vi "Waveform simulator.vi"(1 "Waveform Parameters":T1) -> ()   [LabVIEW 2015]
uses:
  <vilib>/imath/engines/lvmath2/RunTimeEngine/Managers/WorkSpace/UID Generator.vi
  <vilib>/imath/engines/lvmath2/RunTimeEngine/LocalVariableDefStatement/MC_LocalVariableDefStatement_Display.vi
  <vilib>/imath/engines/lvmath2/RunTimeEngine/RunTimeType/NIMS_RunTimeType_From StrictType (excl LVString).vi
  <vilib>/imath/engines/lvmath2/RunTimeEngine/RangeToken/NIMS_Range.vi
  <vilib>/imathl/engines/lvmath/Functions/Error Handling/Create Error.vi
  <vilib>/imath/engines/lvmath2/RunTimeEngine/BuiltInFunctions/linramp/NIMS_linramp.vi
  <vilib>/imath/engines/lvmath2/RunTimeEngine/BuiltInFunctions/gensignal/NIMS_gensignal(str,RS,RS,RS).vi
  <vilib>/imath/engines/lvmath2/RunTimeEngine/BuiltInFunctions/transpose/NIMS_transpose(GV).vi
  <vilib>/imath/engines/lvmath2/RunTimeEngine/ArithmeticOperatorToken/NIMS_ArithmeticOperator_plus.vi
  <vilib>/imath/engines/lvmath2/RunTimeEngine/VariableToken/NIMS_VariableToken_CondDefined.vi
  <vilib>/imath/engines/lvmath2/RunTimeEngine/Managers/SymbolTable/Clear UID.vi
  <vilib>/imath/engines/lvmath2/RunTimeEngine/Managers/SymbolTable/NIMS_WorkSpace.lvlib
  <vilib>/imath/engines/lvmath/Functions/Error Handling/MergeErrorsWrapper.vi
  <vilib>/imath/engines/lvmath2/RunTimeEngine/NodeEndStatement/NIMS_NodeEndStatement_Output.vi
  <vilib>/imath/engines/lvmath2/RunTimeEngine/ErrorHandling/NIMS_Finalize Error.vi
panel:
  in  "Digitizing Parameters":T2
  out "XY Graph":cluster{"t":dbl[], "x":dbl[]}(graph)
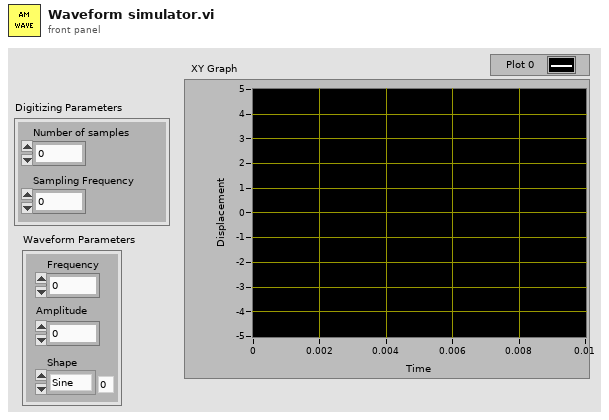
[diagram p1: front panel]
types:
  T1 = cluster{"Frequency":dbl, "Amplitude":dbl, "Shape":enum16{"Sine", "Cosine", "DC Level", "Square", "User Defined"}}
  T2 = cluster{"Number of samples":dbl, "Sampling Frequency":dbl}
  T3 = enum16{"Sine", "Cosine", "DC Level", "Square", "User Defined"}
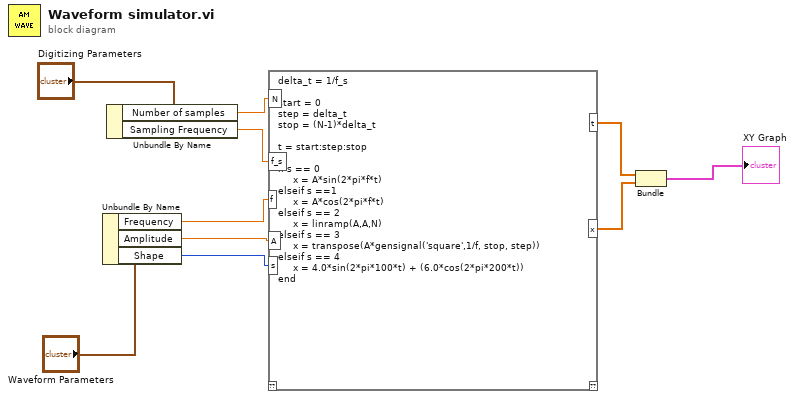
[diagram p0: block diagram]
diagram:
  n1 = Unbundle By Name("Waveform Parameters") -> ("Frequency"=w4:dbl, "Amplitude"=w3:dbl, "Shape"=w2:T3)
  n2 = Unbundle By Name("Digitizing Parameters") -> ("Number of samples"=w7:dbl, "Sampling Frequency"=w6:dbl)
  n3 = mathscript code="delta_t = 1/f_s\n\nstart = 0\nstep = delta_t\nstop = (N-1)*delta_t\n\nt = start:step:stop\n\nif s == 0\n     x = A*sin(2*pi*f*t)\nelseif s ==1\n     x = A*cos(2*pi*f*t)   \nelseif s == 2\n     x = linramp(A,A,N)\nelseif s == 3\n     x = transpose(A*gensignal('square',1/f, stop, step))\nelseif s == 4\n     x = 4.0*sin(2*pi*100*t) + (6.0*cos(2*pi*200*t))\nend"("N"=w7, "f_s"=w6, "f"=w4, "A"=w3, "s"=w2) -> ("x"=w10:dbl[], "t"=w9:dbl[])  [unwired: 1 in, 1 out]
  n4 = Bundle("t"=w9, "x"=w10) -> (→"XY Graph":cluster{"t":dbl[], "x":dbl[]})  [unwired: 1 in]
